vi "Humaniod_Robot_Control.vi"() -> ()   [LabVIEW 2019]
uses:
  <vilib>/Instr/_visa.llb/VISA Configure Serial Port (Instr).vi
panel:
  out "Numeric 18":dbl
  out "Numeric 17":dbl
  out "Numeric 16":dbl
  out "Numeric 15":dbl
  out "Numeric 14":dbl
  out "Numeric 13":dbl
  out "Numeric 12":dbl
  out "Numeric 11":dbl
  out "Numeric 10":dbl
  out "Numeric 9":dbl
  out "Numeric 8":dbl
  out "Numeric 7":dbl
  out "Numeric 6":dbl
  out "Numeric 5":dbl
  out "Numeric 4":dbl
  out "Numeric 3":dbl
  out "Numeric 2":dbl
  out "Numeric":dbl
  out "Title":string
  out "Read String":string
  in  "VISA resource name":refnum<visa-resource-name>
  in  "STOP":bool
  in  "17.RIGHT  THIGH YAW":dbl(slide) scale=200.0..600.0
  in  "16.LEFT THIGH YAW":dbl(slide) scale=200.0..600.0
  in  "15.RIGHT ELBOW ROLL":dbl(slide) scale=200.0..600.0
  in  "14.RIGHT SHOLDER ROLL":dbl(slide) scale=100.0..600.0
  in  "13.RIGHT  SHOULDER PITCH":dbl(slide) scale=200.0..600.0
  in  "12.RIGHT THIGH ROLL":dbl(slide) scale=200.0..500.0
  in  "11.RIGHT THIGH PITCH":dbl(slide) scale=200.0..600.0
  in  "10.RIGHT  KNEE PITCH":dbl(slide) scale=200.0..500.0
  in  "9.RIGHT FOOT  PITCH":dbl(slide) scale=200.0..600.0
  in  "8.RIGHT FOOT ROLL":dbl(slide) scale=200.0..400.0
  in  "7.LEFT FOOT ROLL":dbl(slide) scale=200.0..400.0
  in  "6.LEFT FOOT  PITCH":dbl(slide) scale=200.0..600.0
  in  "5.LEFT  KNEE PITCH":dbl(slide) scale=250.0..500.0
  in  "4.LEFT THIGH PITCH":dbl(slide) scale=200.0..500.0
  out "Write String":string
  in  "3.LEFT THIGH ROLL":dbl(slide) scale=300.0..500.0
  in  "2.LEFT  SHOULDER PITCH":dbl(slide) scale=200.0..600.0
  in  "1.LEFT SHOLDER ROLL":dbl(slide) scale=100.0..600.0
  in  "0.LEFT ELBOW ROLL":dbl(slide) scale=200.0..600.0
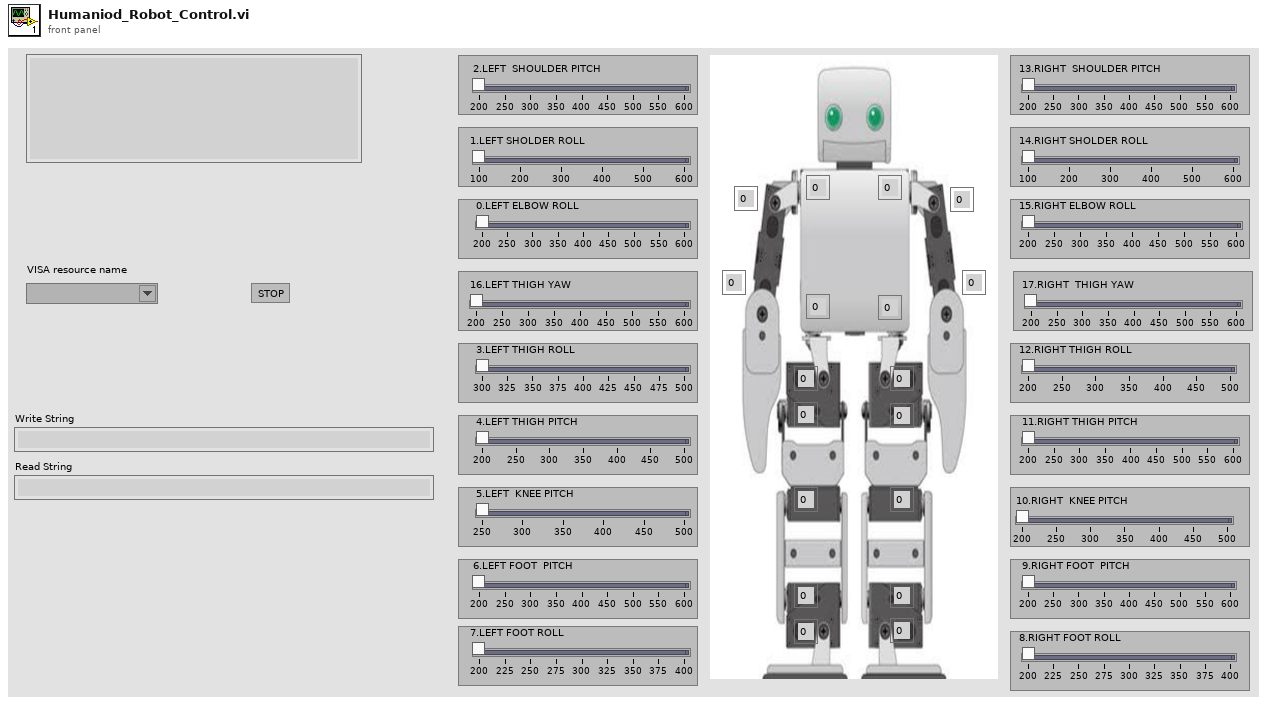
[diagram p1: front panel]
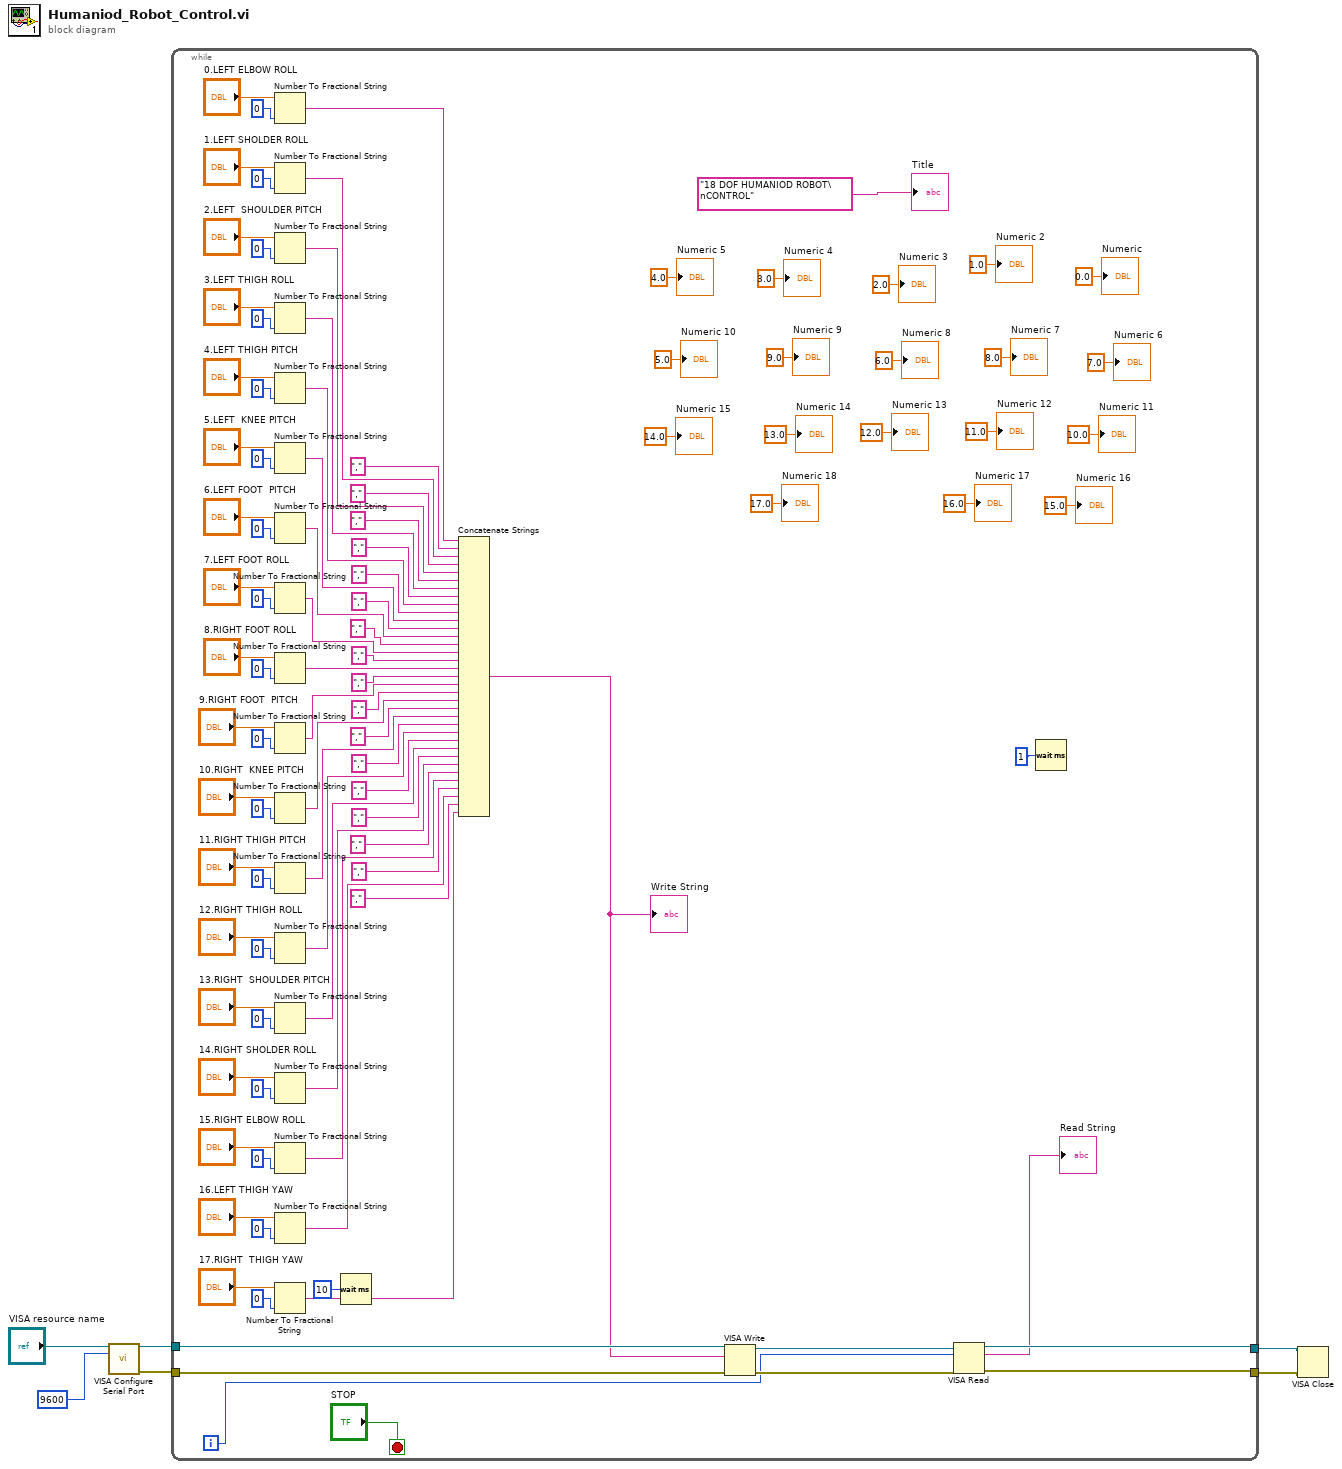
[diagram p0: block diagram]
diagram:
  n1 = call-poly "VISA Configure Serial Port"("VISA resource name"="VISA resource name", "baud rate (9600)"=u32 9600) -> ("VISA resource name out"=w4:refnum<visa-resource-name>, "error out"=w3:errorcluster)  [unwired: 12 in]
  n2 = while {
    tunnel: w4 -> [w106]
    tunnel: w3 -> [w105]
    tunnel: [w30] -> w2
    tunnel: [w28] -> w1
    i -> [w27]
    stop <- "STOP" stop-if-true
    n3 = Number To Fractional String(number="0.LEFT ELBOW ROLL", precision (6)=i16 0) -> (F-format string=w73:string)  [unwired: 2 in]
    n4 = Number To Fractional String(number="1.LEFT SHOLDER ROLL", precision (6)=i16 0) -> (F-format string=w74:string)  [unwired: 2 in]
    n5 = Number To Fractional String(number="2.LEFT  SHOULDER PITCH", precision (6)=i16 0) -> (F-format string=w75:string)  [unwired: 2 in]
    n6 = Number To Fractional String(number="3.LEFT THIGH ROLL", precision (6)=i16 0) -> (F-format string=w76:string)  [unwired: 2 in]
    n7 = Number To Fractional String(number="4.LEFT THIGH PITCH", precision (6)=i16 0) -> (F-format string=w81:string)  [unwired: 2 in]
    n8 = Number To Fractional String(number="5.LEFT  KNEE PITCH", precision (6)=i16 0) -> (F-format string=w82:string)  [unwired: 2 in]
    n9 = Number To Fractional String(number="6.LEFT FOOT  PITCH", precision (6)=i16 0) -> (F-format string=w83:string)  [unwired: 2 in]
    n10 = Number To Fractional String(number="7.LEFT FOOT ROLL", precision (6)=i16 0) -> (F-format string=w84:string)  [unwired: 2 in]
    n11 = Number To Fractional String(number="8.RIGHT FOOT ROLL", precision (6)=i16 0) -> (F-format string=w89:string)  [unwired: 2 in]
    n12 = Number To Fractional String(number="9.RIGHT FOOT  PITCH", precision (6)=i16 0) -> (F-format string=w90:string)  [unwired: 2 in]
    n13 = Number To Fractional String(number="10.RIGHT  KNEE PITCH", precision (6)=i16 0) -> (F-format string=w91:string)  [unwired: 2 in]
    n14 = Number To Fractional String(number="11.RIGHT THIGH PITCH", precision (6)=i16 0) -> (F-format string=w92:string)  [unwired: 2 in]
    n15 = Number To Fractional String(number="12.RIGHT THIGH ROLL", precision (6)=i16 0) -> (F-format string=w99:string)  [unwired: 2 in]
    n16 = Number To Fractional String(number="13.RIGHT  SHOULDER PITCH", precision (6)=i16 0) -> (F-format string=w100:string)  [unwired: 2 in]
    n17 = Number To Fractional String(number="14.RIGHT SHOLDER ROLL", precision (6)=i16 0) -> (F-format string=w101:string)  [unwired: 2 in]
    n18 = Number To Fractional String(number="15.RIGHT ELBOW ROLL", precision (6)=i16 0) -> (F-format string=w102:string)  [unwired: 2 in]
    n19 = Number To Fractional String(number="16.LEFT THIGH YAW", precision (6)=i16 0) -> (F-format string=w103:string)  [unwired: 2 in]
    n20 = Number To Fractional String(number="17.RIGHT  THIGH YAW", precision (6)=i16 0) -> (F-format string=w104:string)  [unwired: 2 in]
    n21 = Wait (ms)(milliseconds to wait=u32 10) -> ()  [unwired: 1 out]
    n22 = Concatenate Strings(w73, ",", w74, ",", w75, ",", w76, ",", w81, ",", w82, ",", w83, ",", w84, ",", w89, ",", w90, ",", w91, ",", w92, ",", w99, ",", w100, ",", w101, ",", w102, ",", w103, ",", w104) -> (w33:string)
    "Write String" <- w33
    n23 = VISA Write(VISA resource name=w106, write buffer=w33, error in (no error)=w105) -> (VISA resource name out=w31:refnum<visa-resource-name>, error out=w29:errorcluster)  [unwired: 1 out]
    n24 = VISA Read(VISA resource name=w31, byte count=w27, error in (no error)=w29) -> (VISA resource name out=w30:refnum<visa-resource-name>, read buffer=→"Read String":string, error out=w28:errorcluster)  [unwired: 1 out]
    n25 = Wait (ms)(milliseconds to wait=u32 1) -> ()  [unwired: 1 out]
    "Title" <- "18 DOF HUMANIOD ROBOT\nCONTROL" ("Title")
    "Numeric" <- 0.0 ("Numeric")
    "Numeric 2" <- 1.0 ("Numeric 2")
    "Numeric 3" <- 2.0 ("Numeric 3")
    "Numeric 4" <- 3.0 ("Numeric 4")
    "Numeric 5" <- 4.0 ("Numeric 5")
    "Numeric 6" <- 7.0 ("Numeric 6")
    "Numeric 7" <- 8.0 ("Numeric 7")
    "Numeric 8" <- 6.0 ("Numeric 8")
    "Numeric 9" <- 9.0 ("Numeric 9")
    "Numeric 10" <- 5.0 ("Numeric 10")
    "Numeric 11" <- 10.0 ("Numeric 11")
    "Numeric 12" <- 11.0 ("Numeric 12")
    "Numeric 13" <- 12.0 ("Numeric 13")
    "Numeric 14" <- 13.0 ("Numeric 14")
    "Numeric 16" <- 15.0 ("Numeric 16")
    "Numeric 18" <- 17.0 ("Numeric 18")
    "Numeric 17" <- 16.0 ("Numeric 17")
    "Numeric 15" <- 14.0 ("Numeric 15")
  }
  n26 = VISA Close(VISA resource name=w2, error in (no error)=w1) -> ()  [unwired: 1 out]
